vi "Cuddle.vi"(8 "error in (no error)":errorcluster, 11 "Baby in":refnum<class "Baby.lvclass">) -> (0 "error out":errorcluster, 3 "Baby out":refnum<class "Baby.lvclass">)   [LabVIEW 2009, in "Baby.lvclass"]
doc: "Cuddle with Baby until she falls asleep."
uses:
  Baby.lvclass
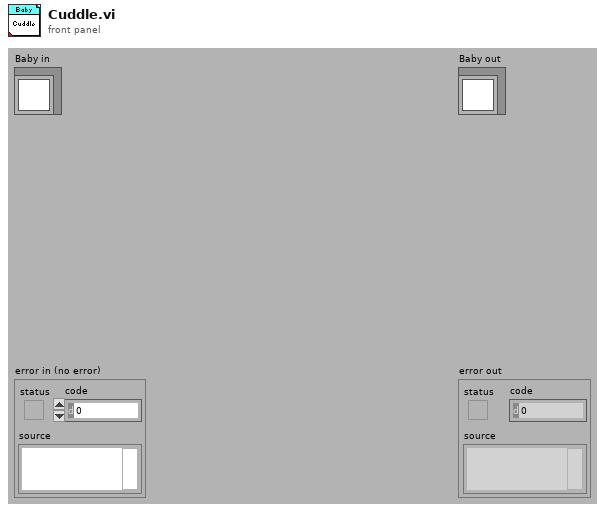
[diagram p1: front panel]
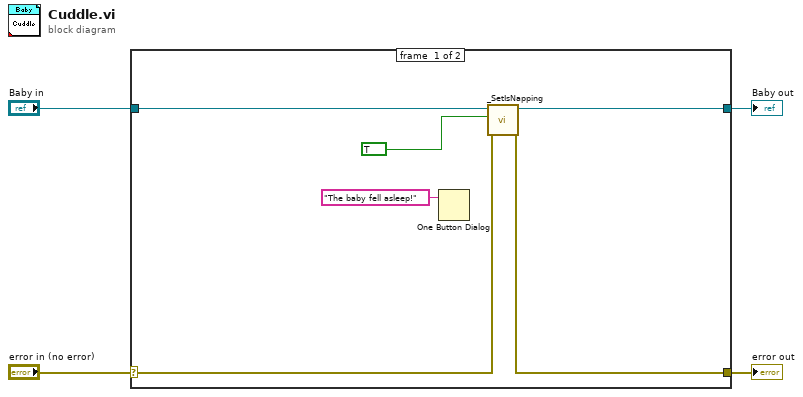
[diagram p0: block diagram]
diagram:
  n1 = case shown="No Error" "error in (no error)" {
    selector: "error in (no error)" -> [w7 w12]
    tunnel: [w6 w12] -> w3
    tunnel: [w8 w11] -> w1
    tunnel: "Baby in" -> [w9 w11]
    frame #0 {
      n2 = One Button Dialog(message="The baby fell asleep!") -> ()  [unwired: 1 in, 1 out]
      n3 = call "_SetIsNapping.vi"("error in (no error)"=w7, "IsNapping (F)"=TRUE ("IsAsleep"), "Baby in"=w9) -> ("error out"=w6:errorcluster, "Baby out"=w8:refnum<class "Baby.lvclass">)  [unwired: 7 in]
    }
    frame #1 {
    }
  }
  "error out" <- w3
  "Baby out" <- w1
